vi "运维调试_氨氮.vi"() -> ()   [LabVIEW 2016, in "斯坦道氨氮.lvlib"]
uses:
  <vilib>/Utility/miscctls.llb/LVPointTypeDef.ctl
  <vilib>/Utility/config.llb/NI_LVConfig.lvlib
  <vilib>/ptbypt/NI_PtbyPt.lvlib
panel:
  in  "模块启用":bool
  in  "串口设置":bool
  in  "备用系数一键写入":bool
  in  "公式一键写入":bool
  in  "流程路径":path=path "C:/Users/STD/Documents/斯坦道流程文件/流程.xml"
  in  "曲线模型":cluster{"X^2":dbl, "X":dbl, "B":dbl}(xcontrol)
  out "字符串":string
  in  "质控参数设置":bool
  in  "自动测试量程配置":T1
  out "温度2":sgl
  out "温度1":sgl
  out "ADC":sgl
  out "固件版本号":string
  in  "数组":string[](array[string])
  in  "备用系数写入":bool
  in  "备用系数读取":bool
  in  "备用系数":T2
  in  "量程切换阈值写入":bool
  in  "量程切换阈值读取":bool
  in  "量程切换阈值":cluster{"阈值":dbl, "标液浓度":dbl}
  in  "参数下拉列表":enum16{"总磷", "总氮", "氨氮"}(ring)=enum."氨氮"
  in  "量程下拉列表":enum16{"低量程", "高量程"}(ring)
  in  "测量模式下拉列表":enum16{"水样测量", "零点核查", "跨度核查", "标样核查", "加标回收"}(ring)
  in  "公式":cluster{"X^2":dbl, "X":dbl, "b":dbl}
  in  "写公式":bool
  in  "读公式":bool
  in  "返回":bool
  in  "设置":bool
  out "序列号":string="序列号"
  out "测量数据":T3(xcontrol)
  out "集成报警信息":string
  out "定时启动":bool
  out "运行状态":T4(xcontrol)
  in  "停止":bool
  in  "手动启动":bool
  in  "单步测试":bool
  in  "总磷氨氮调试":u16[](xcontrol)
  out "F3":sgl format="%#.6f"
  out "F2":sgl format="%#.6f"
  out "F1":sgl format="%#.6f"
  out "F0":sgl format="%#.6f"
  out "多列列表框":i32(listbox)
  # "参数设置"
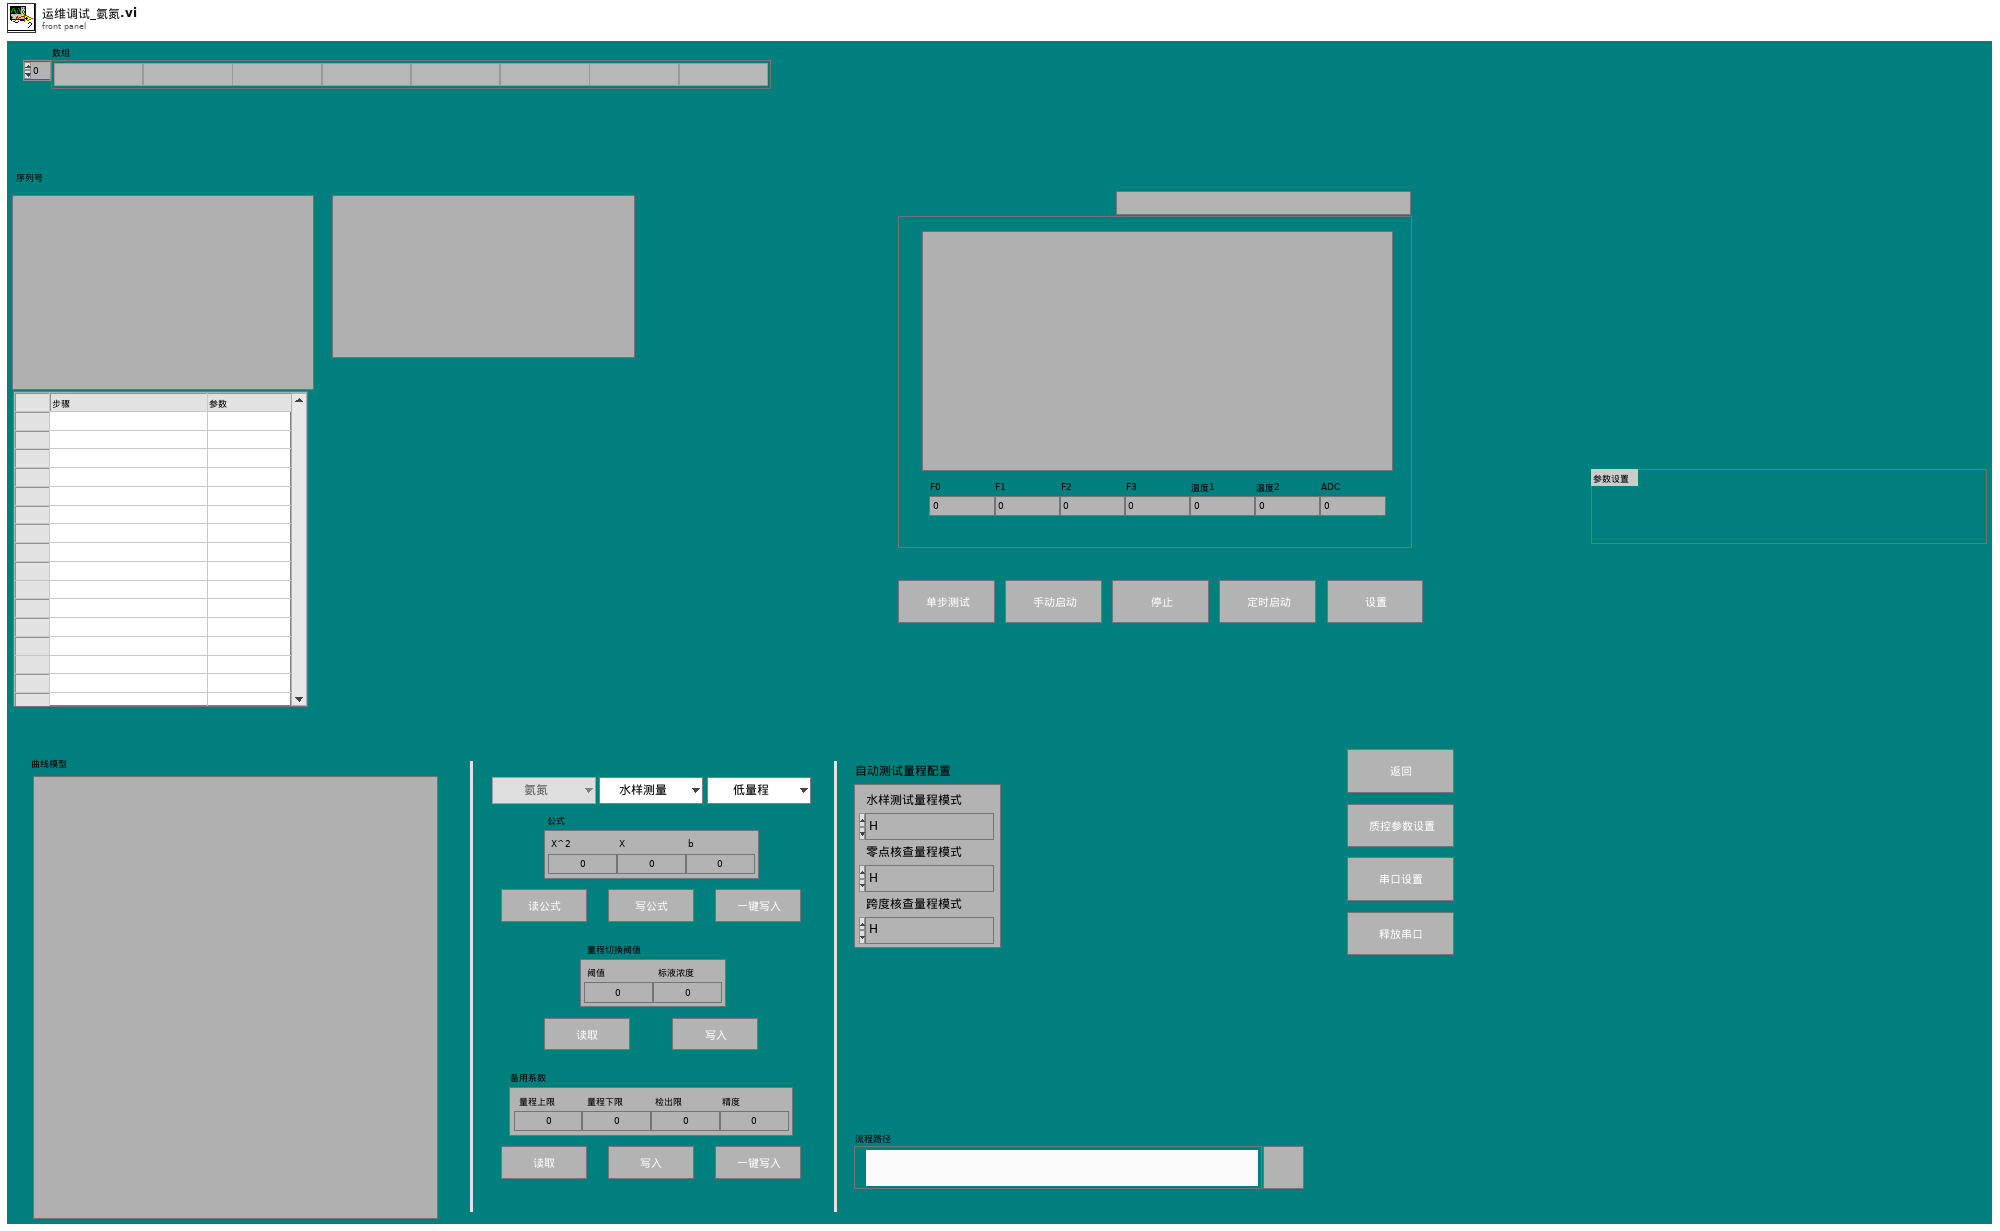
[diagram p1: front panel]
types:
  T1 = cluster{"水样测试量程模式":enum16{"H", "L", "AUTO"}, "空白核查量程模式":enum16{"H", "L", "AUTO"}, "跨度核查量程模式":enum16{"H", "L", "AUTO"}}
  T2 = cluster{"量程上限":dbl, "量程下限":dbl, "检出限":dbl, "精度":dbl}
  T3 = cluster{"flowid":u16, "测量精度":u16, "测量数据区":cluster{"因子编码":u32, "单位":u16, "标样参考值":sgl, "水样数据时间":timestamp, "水样实测值":sgl, "水样数据标识":string, "标样数据时间":timestamp, "标样实测值":sgl, "标样数据标识":string, "空白数据时间":timestamp, "空白实测值":sgl, "空白数据标识":string, "零点核查数据时间":timestamp, "零点核查实测值":sgl, "零点核查数据标识":string, "跨度核查数据时间":timestamp, "跨度核查实测值":sgl, "跨度核查数据标识":string, "加标回收数据时间":timestamp, "加标回收实测值":sgl, "加标回收数据标识":string, "平行样数据时间":timestamp, "平行样实测值":sgl, "平行样数据标识":string, "F0":sgl, "F1":sgl, "F2":sgl, "F3":sgl, "F4":sgl, "F5":sgl, "F6":sgl, "F7":sgl, "温度":sgl, "湿度":sgl, "X值":sgl}}
  T4 = cluster{"系统时间":timestamp, "工作状态":enum16{"空闲", "水样测试", "标样核查", "零点核查", "跨度核查", "空白测试", "平行样测试", "加标回收", "空白校准", "标样校准", "初始化（清洗）"}, "测量模式":enum16{"待机", "连续模式", "周期模式", "定点模式", "受控模式", "手动模式"}, "告警代码":enum16{"无告警", "缺试剂告警", "缺水样告警", "缺蒸馏水告警", "缺标液告警", "仪表漏液告警", "标定异常告警", "超量程告警", "加热异常", "低试剂预警", "超上限告警", "超下限告警", "仪表内部其他异常", "滴定异常告警", "电极异常告警", "量程切换告警", "参数设置告警", "PH电极电位异常", "电导率电极异常", "浊度光度异常", "溶解氧电极异常", "溶解氧光强异常", "温度异常告警", "PH异常告警", "溶解氧异常告警", "电导率异常告警", "浊度异常告警", "叶绿素异常告警", "藻密度异常告警", "蓝绿藻异常告警", "ORP异常告警", "氨氮异常告警", "清洁刷异常告警", "SD卡异常告警", "蓝牙异常告警", "Wifi异常告警", "流程异常告警"}, "故障代码":enum16{"无故障", "电机故障", "温度故障", "通讯故障", "滴定故障"}, "日志代码":u16, "软件版本":u16, "F0":sgl, "F1":sgl, "F2":sgl, "F3":sgl, "T":sgl, "H":sgl, "id":u16, "flowid":u16, "量程":u16, "总磷控温温度1":sgl, "营养盐控温温度2":sgl, "ADC":sgl}
  T5 = enum16{"启动测量", "标样核查", "零点核查", "跨度核查", "空白测试", "平行样测试", "加标回收", "空白校准", "标样校准", "初始化（清洗）", "停止测试", "仪器重启", "校时", "模式设置", "测量间隔设置"}
  T6 = cluster{"控制命令":enum16{"启动测量", "标样核查", "零点核查", "跨度核查", "空白测试", "平行样测试", "加标回收", "空白校准", "标样校准", "初始化（清洗）", "停止测试", "仪器重启", "校时", "模式设置", "测量间隔设置"}, "周期设置类型":enum16{"定点启动", "间隔启动"}, "定时功能启用":bool, "定时间隔":dbl, "24H周期设置":bool[], "零点核查时间":u16, "跨度核查时间":u16, "质控频次":enum16{"关闭", "每天", "星期一", "星期二", "星期三", "星期四", "星期五", "星期六", "星期日"}}
  T7 = enum16{"关闭", "每天", "星期一", "星期二", "星期三", "星期四", "星期五", "星期六", "星期日"}
  T8 = typedef "LVDateTimeRec.ctl" = cluster{"秒数的小数部分":dbl, "秒":i32, "分":i32, "时":i32, "日":i32, "月":i32, "年":i32, "天数（周）":i32, "天数（年）":i32, "DST":i32}
  T9 = enum16{"空闲", "水样测试", "标样核查", "零点核查", "跨度核查", "空白测试", "平行样测试", "加标回收", "空白校准", "标样校准", "初始化（清洗）"}
  T10 = enum32{"Bad", "Idle", "Run top level", "Running"}
  T11 = typedef "LVPointTypeDef.ctl" = cluster{"Horizontal":i16, "Vertical":i16}
  T12 = cluster{"因子编码":u32, "单位":u16, "标样参考值":sgl, "水样数据时间":timestamp, "水样实测值":sgl, "水样数据标识":string, "标样数据时间":timestamp, "标样实测值":sgl, "标样数据标识":string, "空白数据时间":timestamp, "空白实测值":sgl, "空白数据标识":string, "零点核查数据时间":timestamp, "零点核查实测值":sgl, "零点核查数据标识":string, "跨度核查数据时间":timestamp, "跨度核查实测值":sgl, "跨度核查数据标识":string, "加标回收数据时间":timestamp, "加标回收实测值":sgl, "加标回收数据标识":string, "平行样数据时间":timestamp, "平行样实测值":sgl, "平行样数据标识":string, "F0":sgl, "F1":sgl, "F2":sgl, "F3":sgl, "F4":sgl, "F5":sgl, "F6":sgl, "F7":sgl, "温度":sgl, "湿度":sgl, "X值":sgl}
  T13 = typedef "NI_LVConfig.lvlib/Config Data RefNum.ctl" = refnum<k1>
  T14 = cluster{"启动模式":enum16{"跨度核查", "水样测量", "空白核查", "标样核查", "加标回收"}, "启动参数":u16, "量程":enum16{"低量程", "高量程"}}
  T15 = cluster{"时间标识":timestamp, "设备":string, "日志信息":string, "流程参数":string}
  T16 = cluster{"时间标识":timestamp, "设备":string, "日志信息":string}
  T17 = enum16{"无告警", "缺试剂告警", "缺水样告警", "缺蒸馏水告警", "缺标液告警", "仪表漏液告警", "标定异常告警", "超量程告警", "加热异常", "低试剂预警", "超上限告警", "超下限告警", "仪表内部其他异常", "滴定异常告警", "电极异常告警", "量程切换告警", "参数设置告警", "PH电极电位异常", "电导率电极异常", "浊度光度异常", "溶解氧电极异常", "溶解氧光强异常", "温度异常告警", "PH异常告警", "溶解氧异常告警", "电导率异常告警", "浊度异常告警", "叶绿素异常告警", "藻密度异常告警", "蓝绿藻异常告警", "ORP异常告警", "氨氮异常告警", "清洁刷异常告警", "SD卡异常告警", "蓝牙异常告警", "Wifi异常告警", "流程异常告警"}
  T18 = typedef "LVRowAndColumnUnsignedTypeDef.ctl" = cluster{"Row":u32, "Column":u32}
  T19 = cluster{"站号":u16, "量程切换":enum32{"H", "L", "AUTO"}, "控制命令":enum16{"启动测量", "标样核查", "零点核查", "跨度核查", "空白测试", "平行样测试", "加标回收", "空白校准", "标样校准", "初始化（清洗）", "停止测试", "仪器重启", "校时", "模式设置", "测量间隔设置"}, "模式设置":enum16{"待机", "连续模式", "周期模式", "定点模式", "受控模式", "手动模式"}, "测量间隔":u16}
  T20 = cluster{"氨氮跨度值":dbl, "氨氮零点标准液浓度":dbl, "氨氮跨度标准液浓度":dbl, "氨氮标准液标准浓度":dbl}
  T21 = cluster{"确定":bool, "跨度值":dbl, "零点标准液浓度":dbl, "跨度标准液浓度":dbl, "标准液标准浓度":dbl}
  T22 = cluster{"控制命令":enum16{"启动测量", "标样核查", "零点核查", "跨度核查", "空白测试", "平行样测试", "加标回收", "空白校准", "标样校准", "初始化（清洗）", "停止测试", "仪器重启", "校时", "模式设置", "测量间隔设置"}, "周期设置类型":enum16{"定点启动", "间隔启动"}, "定时功能启用":bool, "定时间隔":dbl, "24H周期设置":bool[], "空白核查时间":u16, "跨度核查时间":u16, "质控频次":enum16{"关闭", "每天", "星期一", "星期二", "星期三", "星期四", "星期五", "星期六", "星期日"}}
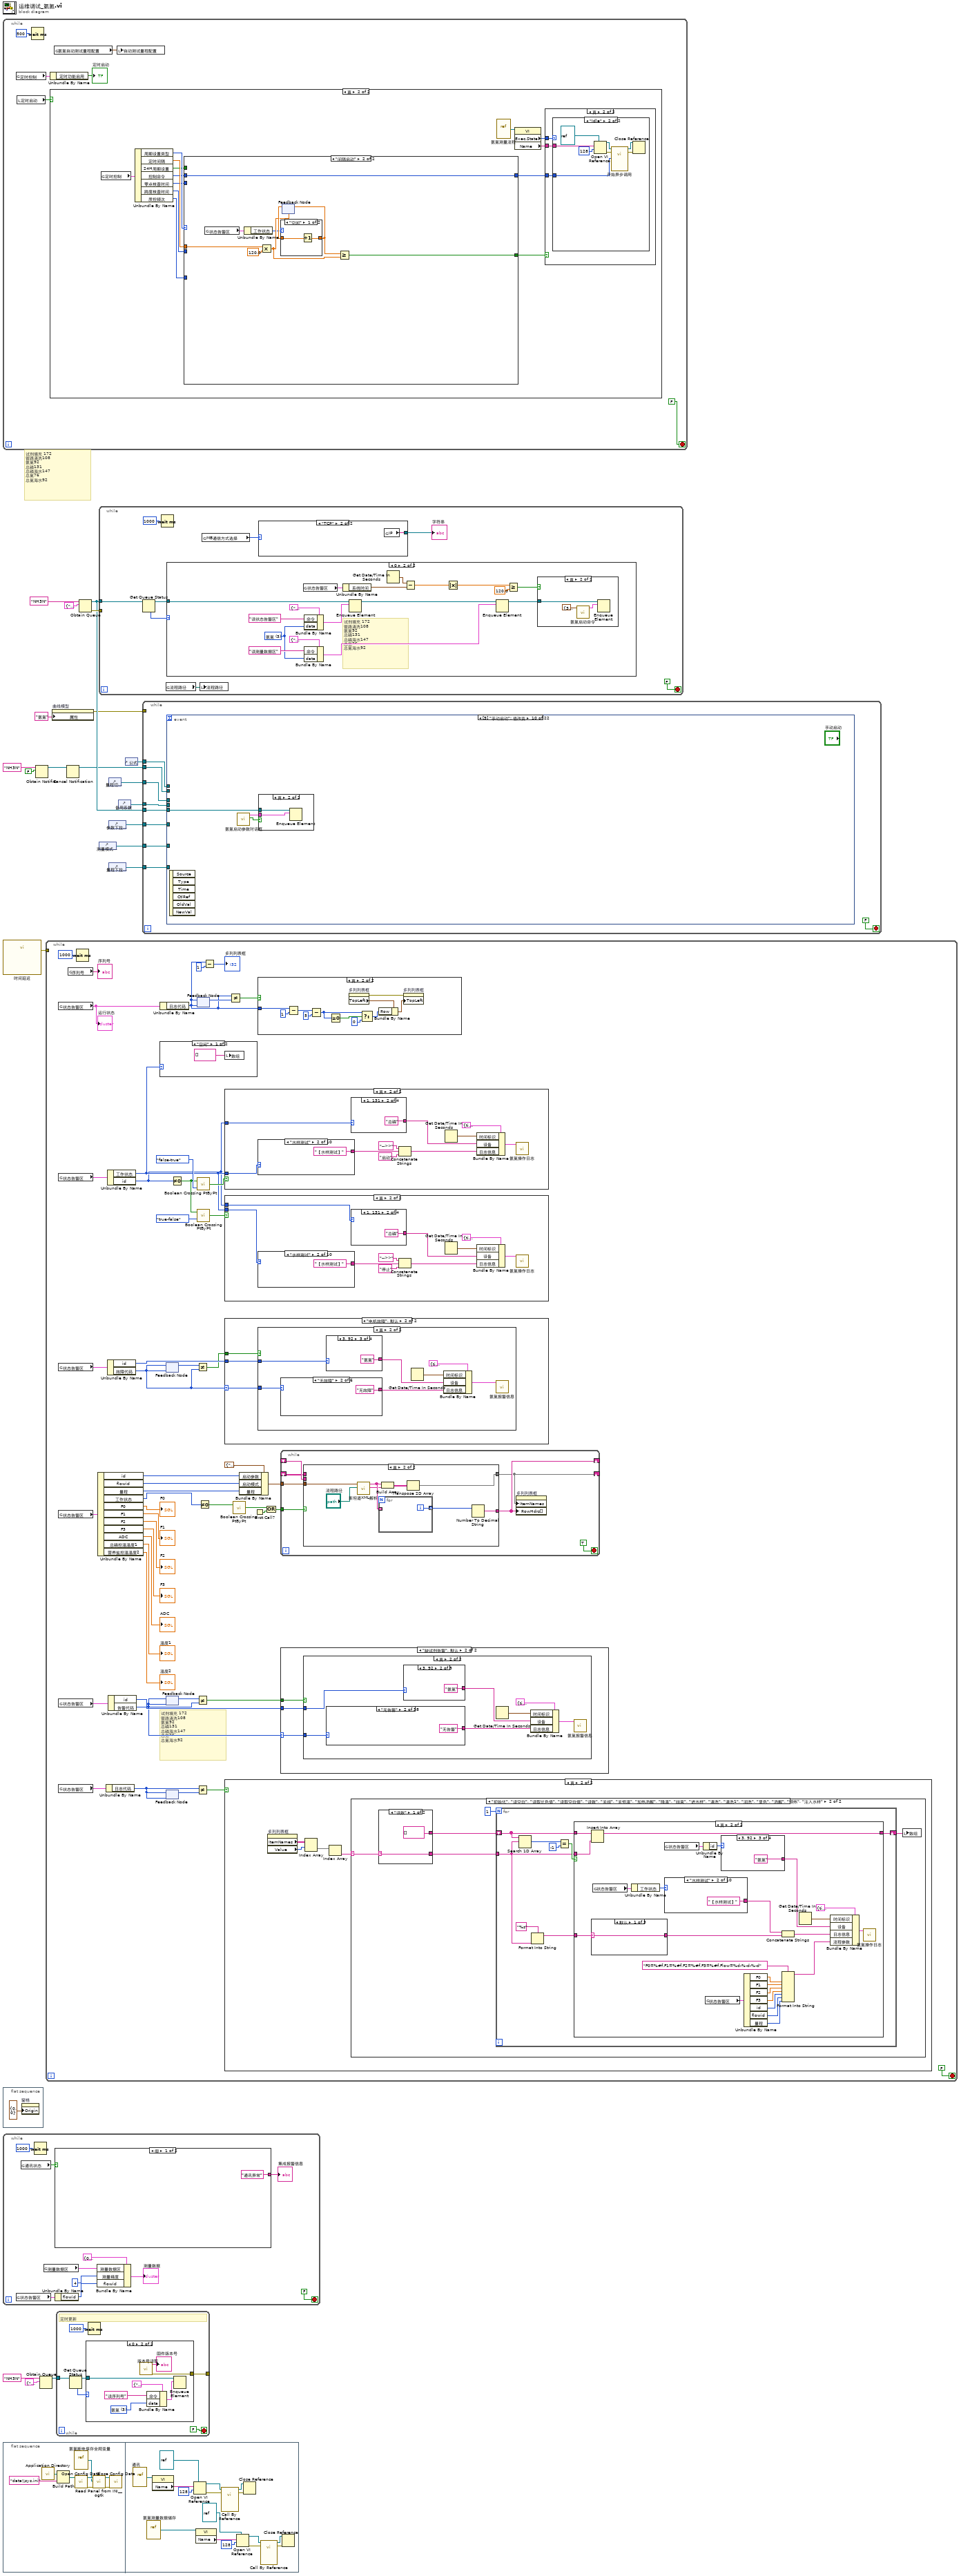
[diagram p0: block diagram]
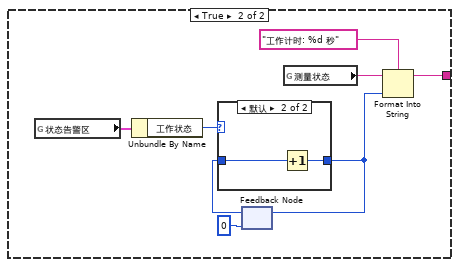
[diagram p3: hidden frame]
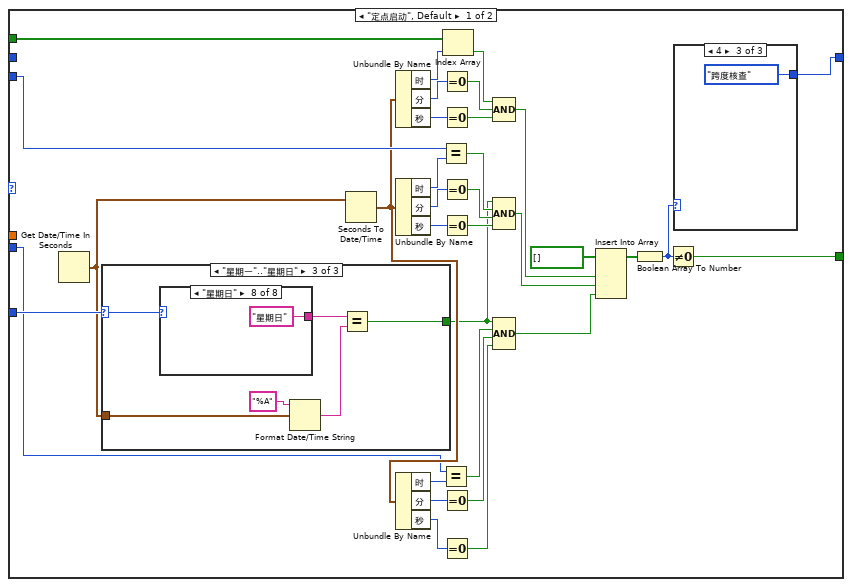
[diagram p8: hidden frame]
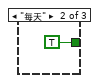
[diagram p10: hidden frame]
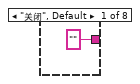
[diagram p11: hidden frame]
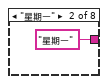
[diagram p12: hidden frame]
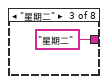
[diagram p13: hidden frame]
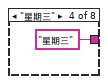
[diagram p14: hidden frame]
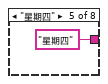
[diagram p15: hidden frame]
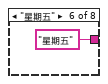
[diagram p16: hidden frame]
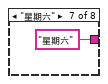
[diagram p17: hidden frame]
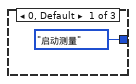
[diagram p18: hidden frame]
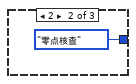
[diagram p19: hidden frame]
diagram:
  # "试剂填充 172 \n管路清洗108\n氨氮92\n总磷131\n总磷海水147\n总氮76\n总氮海水92"
  n1 = while {
    stop <- FALSE stop-if-true
    n2 = global read "氨氮断电保存全局变量.vi" "定时控制"() -> (w22:T6)
    n3 = local read "定时启动"() -> (w24:bool)
    n4 = Wait (ms)(milliseconds to wait=u32 500 ("等待时间（毫秒）")) -> ()  [unwired: 1 out]
    n5 = Unbundle By Name(w22) -> ("定时功能启用"=→"定时启动":bool)
    n6 = case shown="真" w24 {
      frame False {
      }
      frame True {
        n7 = global read "氨氮断电保存全局变量.vi" "定时控制"() -> (w39:T6)
        n8 = Unbundle By Name(w39) -> ("周期设置类型"=w38:enum16{"定点启动", "间隔启动"}, "定时间隔"=w37:dbl, "24H周期设置"=w36:bool[], "控制命令"=w31:T5, "零点核查时间"=w29:u16, "跨度核查时间"=w28:u16, "质控频次"=w27:T7)
        n9 = case shown="\"间隔启动\"" w38 {
          tunnel: w37 -> [_ w108]
          tunnel: w36 -> [w74 _]
          tunnel: [w52 w106] -> w35
          tunnel: w31 -> [_ w104]
          tunnel: [w78 w104] -> w30
          tunnel: w27 -> [w77 _]
          tunnel: w29 -> [w70 _]
          tunnel: w28 -> [w59 _]
          frame "定点启动", Default {
            n10 = Get Date/Time In Seconds() -> (seconds since 1Jan1904=w76:timestamp)
            n11 = case shown="\"星期一\"..\"星期日\"" w77 {
              selector: w77 -> [_ _ w88]
              tunnel: w76 -> [_ _ w89]
              tunnel: [_ TRUE w85] -> w58
              frame "关闭", Default {
              }
              frame "每天" {
              }
              frame "星期一".."星期日" {
                n12 = case shown="\"星期日\"" w88 {
                  tunnel: ["" ("时间格式字符串(%c)") "星期一" ("时间格式字符串(%c)") "星期二" ("时间格式字符串(%c)") "星期三" ("时间格式字符串(%c)") "星期四" ("时间格式字符串(%c)") "星期五" ("时间格式字符串(%c)") "星期六" ("时间格式字符串(%c)") "星期日" ("时间格式字符串(%c)")] -> w87
                  frame "关闭", Default {
                  }
                  frame "星期一" {
                  }
                  frame "星期二" {
                  }
                  frame "星期三" {
                  }
                  frame "星期四" {
                  }
                  frame "星期五" {
                  }
                  frame "星期六" {
                  }
                  frame "星期日" {
                  }
                }
                n13 = Format Date/Time String(time format string (%c)="%A" ("时间格式字符串(%c)"), seconds (now)=w89) -> (date/time string=w86:string)  [unwired: 1 in]
                n14 = Equal?(x=w87, y=w86) -> (x = y?=w85:bool)
              }
            }
            n15 = Seconds To Date/Time(time stamp (now)=w76) -> (date time rec=w60:T8)  [unwired: 1 in]
            n16 = Unbundle By Name(w60) -> ("时"=w83:i32, "分"=w81:i32, "秒"=w82:i32)
            n17 = Unbundle By Name(w60) -> ("时"=w71:i32, "分"=w73:i32, "秒"=w72:i32)
            n18 = Unbundle By Name(w60) -> ("时"=w63:i32, "分"=w61:i32, "秒"=w62:i32)
            n19 = Equal?(x=w70, y=w71) -> (x = y?=w69:bool)
            n20 = Equal?(x=w59, y=w63) -> (x = y?=w64:bool)
            n21 = Equal To 0?(x=w81) -> (x = 0?=w80:bool)
            n22 = Equal To 0?(x=w82) -> (x = 0?=w79:bool)
            n23 = Equal To 0?(x=w73) -> (x = 0?=w68:bool)
            n24 = Equal To 0?(x=w72) -> (x = 0?=w67:bool)
            n25 = Equal To 0?(x=w61) -> (x = 0?=w65:bool)
            n26 = Equal To 0?(x=w62) -> (x = 0?=w66:bool)
            n27 = Index Array(array=w74, index=w83) -> (element=w75:bool)
            n28 = Compound Arithmetic op=AND ("复合运算")(w75, w80, w79) -> (w56:bool)
            n29 = Compound Arithmetic op=AND ("复合运算")(w58, w69, w68, w67) -> (w55:bool)
            n30 = Compound Arithmetic op=AND ("复合运算")(w58, w64, w65, w66) -> (w54:bool)
            n31 = Insert Into Array(array=bool[] [], new element #1=w56, new element #2=w55, new element #3=w54) -> (w53:bool[])  [unwired: 1 in]
            n32 = Boolean Array To Number(Boolean array=w53) -> (number=w51:u32)
            n33 = Not Equal To 0?(x=w51) -> (x != 0?=w52:bool)
            n34 = case shown="4" w51 {
              tunnel: [T5."启动测量" ("控制命令") T5."零点核查" ("控制命令") T5."跨度核查" ("控制命令")] -> w78
              frame 0, Default {
              }
              frame 2 {
              }
              frame 4 {
              }
            }
          }
          frame "间隔启动" {
            n35 = global read "VAR氨氮全局变量.vi" "状态告警区"() -> (w103:T4)
            n36 = Unbundle By Name(w103) -> ("工作状态"=w102:T9)
            n37 = Multiply(x=w108, y=120.0) -> (x*y=w105:dbl)
            n38 = feedback #1(w105) -> (w110:dbl)
            n39 = case shown="\"空闲\"" w102 {
              tunnel: w110 -> [w112 _]
              tunnel: [w111 _] -> w109
              frame "空闲" {
                n40 = Increment(x=w112) -> (x+1=w111:dbl)
              }
              frame "水样测试", Default {
              }
            }
            n41 = feedback-in #1(w109) -> ()
            n42 = Greater Or Equal?(x=w109, y=w105) -> (x >= y?=w106:bool)
          }
        }
        n43 = vi-ref "氨氮测量流程.vi"() -> (w34:refnum<vi>)
        n44 = property class="VI"(reference=w34) -> ("Exec.State"=w33:T10, "Name"=w32:string)  [unwired: 1 in, 2 out]
        n45 = case shown="真" w35 {
          tunnel: w32 -> [_ w42]
          tunnel: w30 -> [_ w41]
          tunnel: w33 -> [_ w40]
          frame False {
          }
          frame True {
            n46 = case shown="\"Idle\"" w40 {
              tunnel: w42 -> [_ w46]
              tunnel: w41 -> [_ w44]
              frame "Bad", Default {
              }
              frame "Idle" {
                n47 = Open VI Reference(type specifier VI Refnum (for type only)=refnum<vi> refnum, vi path=w46, options=128 ("选项")) -> (vi reference=w47:refnum<vi>, error out=w48:errorcluster)  [unwired: 3 in]
                n48 = call-by-ref "开始异步调用"(reference=w47, error in=w48, "控制命令"=w44) -> (reference out=w49:refnum<vi>, error out=w50:errorcluster)  [unwired: 11 in]
                n49 = Close Reference(reference=w49, error in (no error)=w50) -> ()  [unwired: 1 out]
              }
            }
          }
        }
      }
    }
    n50 = global read "氨氮断电保存全局变量.vi" "氨氮自动测试量程配置"() -> (w23:T1)
    n51 = local write "自动测试量程配置"(w23) -> ()
  }
  n52 = call "时间延迟"() -> ("error out"=w10:errorcluster)  [unwired: 11 in]
  n53 = flat-sequence {
    frame #0 {
      n54 = property on="窗格" class="Pane"("Origin"=T11 {"Horizontal"=0, "Vertical"=0} ("原点")) -> ()  [unwired: 2 in, 2 out]
    }
  }
  n55 = while {
    stop <- FALSE stop-if-true
    n56 = global read "VAR氨氮全局变量.vi" "状态告警区"() -> (w119:T4)
    n57 = global read "VAR氨氮全局变量.vi" "通讯状态"() -> (w121:bool)
    n58 = Wait (ms)(milliseconds to wait=u32 1000 ("等待时间（毫秒）")) -> ()  [unwired: 1 out]
    n59 = global read "VAR氨氮全局变量.vi" "测量数据区"() -> (w114:T12)
    n60 = case shown="假" w121 {
      tunnel: ["通讯异常" ("集成报警信息") w126] -> w120
      frame False {
      }
      frame True {
        n61 = global read "VAR氨氮全局变量.vi" "状态告警区"() -> (w132:T4)
        n62 = Unbundle By Name(w132) -> ("工作状态"=w131:T9)
        n63 = feedback #2(0) -> (w129:i32)
        n64 = case shown="默认" w131 {
          tunnel: w129 -> [_ w134]
          tunnel: [_ w133] -> w127
          frame "空闲" {
          }
          frame Default {
            n65 = Increment(x=w134) -> (x+1=w133:i32)
          }
        }
        n66 = feedback-in #2(w127) -> ()
        n67 = global read "VAR氨氮全局变量.vi" "测量状态"() -> (w125:string)
        n68 = Format Into String(format string="工作计时: %d 秒" ("格式字符串"), initial string=w125, w127) -> (resulting string=w126:string)  [unwired: 1 in, 1 out]
      }
    }
    "集成报警信息" <- w120
    n69 = Unbundle By Name(w119) -> ("flowid"=w118:u16)
    n70 = Bundle By Name(cluster=T3 {"flowid"=0, "测量精度"=0, "测量数据区"={"因子编码"=0, "单位"=0, "标样参考值"=0.0, "水样数据时间"=timestamp(0 s since 1904-01-01), "水样实测值"=0.0, "水样数据标识"="", "标样数据时间"=timestamp(0 s since 1904-01-01), "标样实测值"=0.0, "标样数据标识"="", "空白数据时间"=timestamp(0 s since 1904-01-01), "空白实测值"=0.0, "空白数据标识"="", "零点核查数据时间"=timestamp(0 s since 1904-01-01), "零点核查实测值"=0.0, "零点核查数据标识"="", "跨度核查数据时间"=timestamp(0 s since 1904-01-01), "跨度核查实测值"=0.0, "跨度核查数据标识"="", "加标回收数据时间"=timestamp(0 s since 1904-01-01), "加标回收实测值"=0.0, "加标回收数据标识"="", "平行样数据时间"=timestamp(0 s since 1904-01-01), "平行样实测值"=0.0, "平行样数据标识"="", "F0"=0.0, "F1"=0.0, "F2"=0.0, "F3"=0.0, "F4"=0.0, "F5"=0.0, "F6"=0.0, "F7"=0.0, "温度"=0.0, "湿度"=0.0, "X值"=0.0}} ("总氮测量数据"), "测量数据区"=w114, "测量精度"=u16 4, "flowid"=w118) -> (→"测量数据":T3)
  }
  n71 = flat-sequence {
    frame #0 {
      n72 = call <vilib>:"Application Directory.vi"() -> ("Application Directory"=w142:path)
      n73 = Build Path(base path=w142, name or relative path="data\\sys.ini" ("名称或相对路径")) -> (appended path=w140:path)
      n74 = vi-ref "氨氮断电保存全局变量.vi"() -> (w138:refnum<vi>)
      n75 = call <vilib>:"Open Config Data.vi"("configuration file path"=w140) -> ("error out"=w136:errorcluster, "refnum"=w139:T13)  [unwired: 8 in, 1 out]
      n76 = call <userlib>:"Read Panel from INI__ogtk.vi"("error in (no error)"=w136, "VI ref"=w138, "refnum"=w139) -> ("error out"=w135:errorcluster, "refnum out"=w137:T13)  [unwired: 7 in]
      n77 = call <vilib>:"Close Config Data.vi"("error in (no error)"=w135, "refnum"=w137) -> ()  [unwired: 8 in, 2 out]
    }
    frame #1 {
      n78 = vi-ref "通讯.vi"() -> (w158:refnum<vi>)
      n79 = vi-ref "氨氮测量数据储存.vi"() -> (w150:refnum<vi>)
      n80 = property class="VI"(reference=w158) -> ("Name"=w157:string)  [unwired: 1 in, 2 out]
      n81 = Open VI Reference(type specifier VI Refnum (for type only)=refnum<vi> refnum, vi path=w157, options=128 ("选项")) -> (vi reference=w155:refnum<vi>, error out=w153:errorcluster)  [unwired: 3 in]
      n82 = property class="VI"(reference=w150) -> ("Name"=w143:string)  [unwired: 1 in, 2 out]
      n83 = call-by-ref "?"(reference=w155, error in=w153) -> (reference out=w151:refnum<vi>, error out=w152:errorcluster)  [unwired: 12 in]
      n84 = Open VI Reference(type specifier VI Refnum (for type only)=refnum<vi> refnum, vi path=w143, options=128 ("选项")) -> (vi reference=w145:refnum<vi>, error out=w147:errorcluster)  [unwired: 3 in]
      n85 = Close Reference(reference=w151, error in (no error)=w152) -> ()  [unwired: 1 out]
      n86 = call-by-ref "?"(reference=w145, error in=w147) -> (reference out=w149:refnum<vi>, error out=w148:errorcluster)  [unwired: 12 in]
      n87 = Close Reference(reference=w149, error in (no error)=w148) -> ()  [unwired: 1 out]
    }
  }
  n88 = Obtain Notifier(name (unnamed)="NH3N" ("名称（未命名）"), notification data type=FALSE) -> (notifier out=w2:refnum<notifier>)  [unwired: 2 in, 2 out]
  n89 = Obtain Queue(name (unnamed)="NH3N" ("名称（未命名）"), element data type=cluster{"命令":string, "data":variant} {"命令"="", "data"=variant}) -> (queue out=w7:refnum<queue>)  [unwired: 3 in, 2 out]
  n90 = while {
    tunnel: w10 -> [_]
    stop <- FALSE stop-if-true
    # "试剂填充 172 \n管路清洗108\n氨氮92\n总磷131\n总磷海水147\n总氮76\n总氮海水92"
    n91 = global read "VAR氨氮全局变量.vi" "状态告警区"() -> (w192:T4)
    "运行状态" <- w192
    n92 = global read "VAR氨氮全局变量.vi" "状态告警区"() -> (w179:T4)
    n93 = global read "VAR氨氮全局变量.vi" "状态告警区"() -> (w184:T4)
    n94 = global read "VAR氨氮全局变量.vi" "状态告警区"() -> (w200:T4)
    n95 = global read "VAR氨氮全局变量.vi" "状态告警区"() -> (w189:T4)
    n96 = global read "VAR氨氮全局变量.vi" "状态告警区"() -> (w177:T4)
    n97 = global read "VAR氨氮全局变量.vi" "序列号"() -> (→"序列号":string)
    n98 = Wait (ms)(milliseconds to wait=u32 1000 ("等待时间（毫秒）")) -> ()  [unwired: 1 out]
    n99 = Unbundle By Name(w200) -> ("id"=w197:u16, "flowid"=w199:u16, "量程"=w198:u16, "工作状态"=w167:T9, "F0"=→"F0":sgl, "F1"=→"F1":sgl, "F2"=→"F2":sgl, "F3"=→"F3":sgl, "ADC"=→"ADC":sgl, "总磷控温温度1"=→"温度1":sgl, "营养盐控温温度2"=→"温度2":sgl)
    n100 = Unbundle By Name(w177) -> ("日志代码"=w176:u16)
    n101 = Unbundle By Name(w179) -> ("工作状态"=w163:T9, "id"=w162:u16)
    n102 = Unbundle By Name(w184) -> ("id"=w183:u16, "故障代码"=w180:enum16{"无故障", "电机故障", "温度故障", "通讯故障", "滴定故障"})
    n103 = Unbundle By Name(w189) -> ("id"=w188:u16, "告警代码"=w185:T17)
    n104 = Unbundle By Name(w192) -> ("日志代码"=w173:u16)
    n105 = case shown="\"空闲\"" w163 {
      frame "空闲" {
        n106 = local write "数组"(string[] [] ("数组")) -> ()
      }
      frame "水样测试", Default {
      }
    }
    n107 = feedback #3(w180) -> (w181:enum16{"无故障", "电机故障", "温度故障", "通讯故障", "滴定故障"})
    n108 = feedback-in #3(w180) -> ()
    n109 = feedback #4(w185) -> (w186:T17)
    n110 = feedback-in #4(w185) -> ()
    n111 = feedback #5(w176) -> (w178:u16)
    n112 = feedback-in #5(w176) -> ()
    n113 = Not Equal To 0?(x=w162) -> (x != 0?=w160:bool)
    n114 = Not Equal?(x=w181, y=w180) -> (x != y?=w182:bool)
    n115 = Not Equal?(x=w186, y=w185) -> (x != y?=w187:bool)
    n116 = Not Equal?(x=w176, y=w178) -> (x != y?=w175:bool)
    n117 = feedback-in #6(w173) -> ()
    n118 = feedback #6(w173) -> (w205:u16)
    n119 = call <vilib>:"Boolean Crossing PtByPt.vi"("direction"=enum16{"either", "false-true", "true-false"}."false-true", "input"=w160) -> ("crossing"=w164:bool)  [unwired: 1 in]
    n120 = call <vilib>:"Boolean Crossing PtByPt.vi"("direction"=enum16{"either", "false-true", "true-false"}."true-false", "input"=w160) -> ("crossing"=w159:bool)  [unwired: 1 in]
    n121 = Not Equal To 0?(x=w167) -> (x != 0?=w202:bool)
    n122 = Subtract(x=w173, y=1) -> (x-y=→"多列列表框":i32)
    n123 = case shown="真" w164 {
      tunnel: w162 -> [_ w232]
      tunnel: w163 -> [_ w231]
      frame False {
      }
      frame True {
        n124 = case shown="\"水样测试\"" w231 {
          tunnel: [_ "【水样测试】" ("字符串") "【标样核查】" ("字符串") "【零点核查】" ("字符串") "【跨度核查】" ("字符串") "【空白测试】" ("字符串") "【平行样测试】" ("字符串") "【加标回收】" ("字符串") "【空白校准】" ("字符串") "【标样校准】" ("字符串")] -> w236
          frame "空闲", Default {
          }
          frame "水样测试" {
          }
          frame "标样核查" {
          }
          frame "零点核查" {
          }
          frame "跨度核查" {
          }
          frame "空白测试" {
          }
          frame "平行样测试" {
          }
          frame "加标回收" {
          }
          frame "空白校准" {
          }
          frame "标样校准" {
          }
        }
        n125 = case shown="1, 131" w232 {
          tunnel: [_ "总磷" ("table输入") "氨氮" ("table输入") "总氮" ("table输入")] -> w237
          frame Default {
          }
          frame 1, 131 {
          }
          frame 3, 92 {
          }
          frame 2, 76 {
          }
        }
        n126 = Concatenate Strings("-->>" ("字符串"), w236, "启动" ("字符串")) -> (w235:string)
        n127 = Get Date/Time In Seconds() -> (seconds since 1Jan1904=w238:timestamp)
        n128 = Bundle By Name(cluster=T15 {"时间标识"=timestamp(0 s since 1904-01-01), "设备"="", "日志信息"="", "流程参数"=""} ("data in"), "时间标识"=w238, "设备"=w237, "日志信息"=w235) -> (w230:T15)
        n129 = call "氨氮操作日志.vi"("data in"=w230) -> ()  [unwired: 11 in]
      }
    }
    n130 = case shown="真" w159 {
      tunnel: w162 -> [_ w210]
      tunnel: w163 -> [_ w209]
      frame False {
      }
      frame True {
        n131 = case shown="\"水样测试\"" w209 {
          tunnel: [_ "【水样测试】" ("字符串") "【标样核查】" ("字符串") "【零点核查】" ("字符串") "【跨度核查】" ("字符串") "【空白测试】" ("字符串") "【平行样测试】" ("字符串") "【加标回收】" ("字符串") "【空白校准】" ("字符串") "【标样校准】" ("字符串")] -> w214
          frame "空闲", Default {
          }
          frame "水样测试" {
          }
          frame "标样核查" {
          }
          frame "零点核查" {
          }
          frame "跨度核查" {
          }
          frame "空白测试" {
          }
          frame "平行样测试" {
          }
          frame "加标回收" {
          }
          frame "空白校准" {
          }
          frame "标样校准" {
          }
        }
        n132 = case shown="1, 131" w210 {
          tunnel: [_ "总磷" ("table输入") "氨氮" ("table输入") "总氮" ("table输入")] -> w215
          frame Default {
          }
          frame 1, 131 {
          }
          frame 3, 92 {
          }
          frame 2, 76 {
          }
        }
        n133 = Concatenate Strings("-->>" ("字符串"), w214, "停止" ("字符串")) -> (w213:string)
        n134 = Get Date/Time In Seconds() -> (seconds since 1Jan1904=w216:timestamp)
        n135 = Bundle By Name(cluster=T15 {"时间标识"=timestamp(0 s since 1904-01-01), "设备"="", "日志信息"="", "流程参数"=""} ("data in"), "时间标识"=w216, "设备"=w215, "日志信息"=w213) -> (w208:T15)
        n136 = call "氨氮操作日志.vi"("data in"=w208) -> ()  [unwired: 11 in]
      }
    }
    n137 = case shown="\"电机故障\", 默认" w180 {
      selector: w180 -> [_ w320]
      tunnel: w183 -> [_ w321]
      tunnel: w182 -> [_ w319]
      frame "无故障" {
      }
      frame "电机故障", Default {
        n138 = case shown="真" w319 {
          tunnel: w321 -> [_ w328]
          tunnel: w320 -> [_ w323]
          frame False {
          }
          frame True {
            n139 = case shown="\"无故障\"" w323 {
              selector: w323 -> [w330 _ _ _ _ _]
              tunnel: [w329 "无故障" "电机故障" "温度故障" "通讯故障" "滴定故障"] -> w322
              frame Default {
                n140 = Format Into String(format string="%d" ("格式字符串"), initial string="未知" ("工作状态"), w330) -> (resulting string=w329:string)  [unwired: 1 in, 1 out]
              }
              frame "无故障" {
              }
              frame "电机故障" {
              }
              frame "温度故障" {
              }
              frame "通讯故障" {
              }
              frame "滴定故障" {
              }
            }
            n141 = case shown="3, 92" w328 {
              tunnel: [_ "总磷" ("table输入") "氨氮" ("table输入") "总氮" ("table输入")] -> w324
              frame Default {
              }
              frame 1, 131 {
              }
              frame 3, 92 {
              }
              frame 2, 76 {
              }
            }
            n142 = Get Date/Time In Seconds() -> (seconds since 1Jan1904=w325:timestamp)
            n143 = Bundle By Name(cluster=T16 {"时间标识"=timestamp(0 s since 1904-01-01), "设备"="", "日志信息"=""} ("data in"), "时间标识"=w325, "设备"=w324, "日志信息"=w322) -> (w326:T16)
            n144 = call "氨氮报警信息.vi"("data in"=w326) -> ()  [unwired: 10 in, 1 out]
          }
        }
      }
    }
    n145 = case shown="真" w175 {
      frame False {
      }
      frame True {
        n146 = property on="多列列表框" class="MCListbox (严格)"() -> ("ItemNames"=w255:string[][], "Value"=w256:i32)  [unwired: 2 in, 2 out]
        n147 = Index Array(array=w255, index (row)=w256) -> (element=w254:string[])  [unwired: 1 in]
        n148 = Index Array(array=w254) -> (element=w253:string)  [unwired: 1 in]
        n149 = case shown="\"初始化\", \"读空白\", \"读取比色值\", \"读取空白值\", \"读数\", \"关阀\", \"关恒温\", \"加热消解\", \"降温\", \"结束\", \"进水样\", \"清洗\", \"清洗1\", \"润洗\", \"显色\", \"消解\", \"预热\", \"注入水样\"" w253 {
          selector: w253 -> [_ w259]
          frame Default {
          }
          frame "初始化", "读空白", "读取比色值", "读取空白值", "读数", "关阀", "关恒温", "加热消解", "降温", "结束", "进水样", "清洗", "清洗1", "润洗", "显色", "消解", "预热", "注入水样" {
            n150 = case shown="\"读数\"" w259 {
              selector: w259 -> [w263 w265]
              tunnel: [w263 w265] -> w258
              tunnel: [string[] [] ("数组") "数组"] -> w257
              frame "读数" {
              }
              frame Default {
              }
            }
            n151 = for {
              N: 1 -> [_]
              tunnel: w258 -> [w267]
              shift-right: [w266] -> w260
              shift-left: w257 -> [w268]
              n152 = Search 1D Array(1D array=w268, element=w267) -> (index of element=w271:i32)  [unwired: 1 in]
              n153 = Format Into String(format string="%s" ("格式字符串"), w267) -> (resulting string=w272:string)  [unwired: 2 in, 1 out]
              n154 = Equal?(x=w271, y=-1) -> (x = y?=w269:bool)
              n155 = case shown="真" w269 {
                tunnel: w272 -> [_ w280]
                tunnel: w268 -> [w274 w284]
                tunnel: w267 -> [_ w283]
                tunnel: [w274 w282] -> w266
                frame False {
                }
                frame True {
                  n156 = Insert Into Array(array=w284, new element=w283) -> (w282:string[])  [unwired: 1 in]
                  n157 = case shown="默认" w280 {
                    selector: w280 -> [w309 w312 w315]
                    tunnel: [w309 w311 w314] -> w279
                    frame Default {
                    }
                    frame "初始化" {
                      n158 = Concatenate Strings("-->>" ("字符串"), w312) -> (w311:string)
                    }
                    frame "结束" {
                      n159 = Concatenate Strings("-->>" ("字符串"), w315) -> (w314:string)
                    }
                  }
                  n160 = global read "VAR氨氮全局变量.vi" "状态告警区"() -> (w278:T4)
                  n161 = Unbundle By Name(w278) -> ("工作状态"=w277:T9)
                  n162 = global read "VAR氨氮全局变量.vi" "状态告警区"() -> (w299:T4)
                  n163 = case shown="\"水样测试\"" w277 {
                    tunnel: [_ "【水样测试】" ("字符串") "【标样核查】" ("字符串") "【零点核查】" ("字符串") "【跨度核查】" ("字符串") "【空白测试】" ("字符串") "【平行样测试】" ("字符串") "【加标回收】" ("字符串") "【空白校准】" ("字符串") "【标样校准】" ("字符串")] -> w275
                    frame "空闲", Default {
                    }
                    frame "水样测试" {
                    }
                    frame "标样核查" {
                    }
                    frame "零点核查" {
                    }
                    frame "跨度核查" {
                    }
                    frame "空白测试" {
                    }
                    frame "平行样测试" {
                    }
                    frame "加标回收" {
                    }
                    frame "空白校准" {
                    }
                    frame "标样校准" {
                    }
                  }
                  n164 = Unbundle By Name(w299) -> ("id"=w298:u16)
                  n165 = global read "VAR氨氮全局变量.vi" "状态告警区"() -> (w294:T4)
                  n166 = case shown="3, 92" w298 {
                    tunnel: [_ "总磷" ("table输入") "氨氮" ("table输入") "总氮" ("table输入")] -> w296
                    frame Default {
                    }
                    frame 1, 131 {
                    }
                    frame 3, 92 {
                    }
                    frame 2, 76 {
                    }
                  }
                  n167 = Unbundle By Name(w294) -> ("F0"=w291:sgl, "F1"=w290:sgl, "F2"=w289:sgl, "F3"=w288:sgl, "id"=w287:u16, "flowid"=w286:u16, "量程"=w285:u16)
                  n168 = Concatenate Strings(w275, w279) -> (w276:string)
                  n169 = Format Into String(format string="F0=%#f,F1=%#f,F2=%#f,F3=%#f,Flow=%d-%-d-%-d" ("格式字符串"), w291, w290, w289, w288, w287, w286, w285) -> (resulting string=w292:string)  [unwired: 2 in, 1 out]
                  n170 = Get Date/Time In Seconds() -> (seconds since 1Jan1904=w295:timestamp)
                  n171 = Bundle By Name(cluster=T15 {"时间标识"=timestamp(0 s since 1904-01-01), "设备"="", "日志信息"="", "流程参数"=""} ("data in"), "时间标识"=w295, "设备"=w296, "日志信息"=w276, "流程参数"=w292) -> (w297:T15)
                  n172 = call "氨氮操作日志.vi"("data in"=w297) -> ()  [unwired: 11 in]
                }
              }
            }
            n173 = local write "数组"(w260) -> ()
          }
        }
      }
    }
    n174 = Not Equal?(x=w173, y=w205) -> (x != y?=w204:bool)
    n175 = call <vilib>:"Boolean Crossing PtByPt.vi"("input"=w202) -> ("crossing"=w166:bool)  [unwired: 2 in]
    n176 = Bundle By Name(cluster=T14 {"启动模式"=enum."跨度核查", "启动参数"=1, "量程"=enum."低量程"} ("参数簇"), "启动参数"=w197, "启动模式"=w199, "量程"=w198) -> (w191:T14)
    n177 = First Call?() -> (First Call?: T/F=w203:bool)
    n178 = case shown="真" w204 {
      tunnel: w173 -> [_ w415]
      frame False {
      }
      frame True {
        n179 = Subtract(x=w415, y=1) -> (x-y=w413:i32)
        n180 = Subtract(x=w413, y=5) -> (x-y=w417:i32)
        n181 = Greater Or Equal To 0?(x=w417) -> (x >= 0?=w416:bool)
        n182 = property on="多列列表框" class="MCListbox (严格)"() -> (error out=w421:errorcluster, "TopLeft"=w422:T18)  [unwired: 2 in, 1 out]
        n183 = Select(t=w417, s=w416, f=0) -> (s? t:f=w418:i32)
        n184 = Bundle By Name(cluster=w422, "Row"=w418) -> (w423:T18)
        n185 = property on="多列列表框" class="MCListbox (严格)"(error in=w421, "TopLeft"=w423) -> ()  [unwired: 1 in, 2 out]
      }
    }
    n186 = Or(x=w166, y=w203) -> (x .or. y?=w201:bool)
    n187 = while {
      tunnel: w201 -> [w401]
      tunnel: w191 -> [w400]
      shift-right: [w395] -> _
      shift-left: _ -> [w397]
      shift-right: [w396] -> _
      shift-left: _ -> [w398]
      stop <- TRUE stop-if-true
      n188 = case shown="真" w401 {
        tunnel: [w403 w411] -> w396
        tunnel: [w402 w410] -> w395
        tunnel: w400 -> [_ w405]
        tunnel: w398 -> [w403 _]
        tunnel: w397 -> [w402 _]
        frame False {
        }
        frame True {
          n189 = call "斯坦道XML解析.vi"("添加的路径"="流程路径", "参数簇"=w405) -> ("步骤时间"=w406:string[], "步骤名"=w408:string[])  [unwired: 8 in]
          n190 = for {
            tunnel: w408 -> [_] mode=indexing
            tunnel: [w412] -> w409 mode=indexing
            i -> [w412]
          }
          n191 = Build Array(w408, w406) -> (w407:string[][])
          n192 = Transpose 2D Array(2D array=w407) -> (transposed array=w410:string[][])
          n193 = Number To Decimal String(number=w409) -> (decimal integer string=w411:string[])  [unwired: 1 in]
        }
      }
      n194 = property on="多列列表框" class="MCListbox (严格)"("ItemNames"=w395, "RowHdrs[]"=w396) -> ()  [unwired: 2 in, 2 out]
    }
    n195 = case shown="\"缺试剂告警\", 默认" w185 {
      selector: w185 -> [_ w342]
      tunnel: w188 -> [_ w343]
      tunnel: w187 -> [_ w341]
      frame "无告警" {
      }
      frame "缺试剂告警", Default {
        n196 = case shown="真" w341 {
          tunnel: w343 -> [_ w350]
          tunnel: w342 -> [_ w344]
          frame False {
          }
          frame True {
            n197 = case shown="\"无告警\"" w344 {
              selector: w344 -> [w352 _ _ _ _ _ _ _ _ _ _ _ _ _ _ _ _ _ _ _ _ _ _ _ _ _ _ _ _ _ _ _ _ _ _ _ _ _]
              tunnel: [w351 "无告警" "缺试剂告警" "缺水样告警" "缺蒸馏水告警" "缺标液告警" "仪表漏液告警" "标定异常告警" "超量程告警" "加热异常" "低试剂预警" "超上限告警" "超下限告警" "仪表内部其他异常" "滴定异常告警" "电极异常告警" "量程切换告警" "参数设置告警" "PH电极电位异常" "电导率电极异常" "浊度光度异常" "溶解氧电极异常" "溶解氧光强异常" "温度异常告警" "PH异常告警" "溶解氧异常告警" "电导率异常告警" "浊度异常告警" "叶绿素异常告警" "藻密度异常告警" "蓝绿藻异常告警" "ORP异常告警" "氨氮异常告警" "清洁刷异常告警" "SD卡异常告警" "蓝牙异常告警" "WiFi异常告警" "流程异常告警"] -> w345
              frame Default {
                n198 = Format Into String(format string="%d" ("格式字符串"), initial string="未知" ("工作状态"), w352) -> (resulting string=w351:string)  [unwired: 1 in, 1 out]
              }
              frame "无告警" {
              }
              frame "缺试剂告警" {
              }
              frame "缺水样告警" {
              }
              frame "缺蒸馏水告警" {
              }
              frame "缺标液告警" {
              }
              frame "仪表漏液告警" {
              }
              frame "标定异常告警" {
              }
              frame "超量程告警" {
              }
              frame "加热异常" {
              }
              frame "低试剂预警" {
              }
              frame "超上限告警" {
              }
              frame "超下限告警" {
              }
              frame "仪表内部其他异常" {
              }
              frame "滴定异常告警" {
              }
              frame "电极异常告警" {
              }
              frame "量程切换告警" {
              }
              frame "参数设置告警" {
              }
              frame "PH电极电位异常" {
              }
              frame "电导率电极异常" {
              }
              frame "浊度光度异常" {
              }
              frame "溶解氧电极异常" {
              }
              frame "溶解氧光强异常" {
              }
              frame "温度异常告警" {
              }
              frame "PH异常告警" {
              }
              frame "溶解氧异常告警" {
              }
              frame "电导率异常告警" {
              }
              frame "浊度异常告警" {
              }
              frame "叶绿素异常告警" {
              }
              frame "藻密度异常告警" {
              }
              frame "蓝绿藻异常告警" {
              }
              frame "ORP异常告警" {
              }
              frame "氨氮异常告警" {
              }
              frame "清洁刷异常告警" {
              }
              frame "SD卡异常告警" {
              }
              frame "蓝牙异常告警" {
              }
              frame "Wifi异常告警" {
              }
              frame "流程异常告警" {
              }
            }
            n199 = case shown="3, 92" w350 {
              tunnel: ["总磷" ("table输入") "氨氮" ("table输入") "总氮" ("table输入")] -> w346
              frame 1, 131 {
              }
              frame 3, 92 {
              }
              frame 2, 76, Default {
              }
            }
            n200 = Get Date/Time In Seconds() -> (seconds since 1Jan1904=w347:timestamp)
            n201 = Bundle By Name(cluster=T16 {"时间标识"=timestamp(0 s since 1904-01-01), "设备"="", "日志信息"=""} ("data in"), "时间标识"=w347, "设备"=w346, "日志信息"=w345) -> (w348:T16)
            n202 = call "氨氮报警信息.vi"("data in"=w348) -> ()  [unwired: 10 in, 1 out]
          }
        }
      }
    }
  }
  n203 = property on="曲线模型" class="曲线模型 (严格)"("属性"="氨氮" ("调用模块名称属性")) -> (error out=w5:errorcluster)  [unwired: 2 in, 1 out]
  n204 = while {
    tunnel: w7 -> [w428]
    tunnel: [w426] -> _
    stop <- FALSE stop-if-true
    # "定时更新"
    n205 = Get Queue Status(queue=w428) -> (queue out=w425:refnum<queue>, # elements in queue=w424:i32)  [unwired: 2 in, 6 out]
    n206 = case shown="0" w424 {
      tunnel: [_ w431] -> w426
      tunnel: w425 -> [_ w430]
      frame Default {
      }
      frame 0 {
        w434 = u16 3 items=["总磷"=1, "氨氮"=3] ("站号")
        n207 = call "版本号读取.vi"() -> ("error out"=w431:errorcluster, "固件版本号"=→"固件版本号":string)  [unwired: 10 in]
        n208 = Bundle By Name(cluster=cluster{"命令":string, "data":variant} {"命令"="", "data"=variant} ("元素"), "命令"="读序列号", "data"=w434) -> (w433:cluster{"命令":string, "data":variant})
        n209 = Enqueue Element(queue=w430, element=w433) -> ()  [unwired: 2 in, 3 out]
      }
    }
    n210 = Wait (ms)(milliseconds to wait=u32 1000 ("等待时间（毫秒）")) -> ()  [unwired: 1 out]
  }
  n211 = Cancel Notification(0:w2) -> (8:w1:refnum<notifier>)  [unwired: 1 in, 2 out]
  n212 = Obtain Queue(name (unnamed)="NH3N" ("名称（未命名）"), element data type=cluster{"命令":string, "data":variant} {"命令"="", "data"=variant}) -> (queue out=w17:refnum<queue>, error out=w18:errorcluster)  [unwired: 3 in, 1 out]
  n213 = while {
    tunnel: w17 -> [w442]
    tunnel: w18 -> [_]
    stop <- FALSE stop-if-true
    n214 = Get Queue Status(queue=w442) -> (queue out=w438:refnum<queue>, # elements in queue=w437:i32)  [unwired: 2 in, 6 out]
    n215 = Wait (ms)(milliseconds to wait=u32 1000 ("等待时间（毫秒）")) -> ()  [unwired: 1 out]
    n216 = global read "氨氮断电保存全局变量.vi" "流程路径"() -> (w441:path)
    n217 = case shown="0" w437 {
      tunnel: w438 -> [_ w445]
      frame Default {
      }
      frame 0 {
        w454 = u16 3 items=["总磷"=1, "氨氮"=3] ("站号")
        # "试剂填充 172 \n管路清洗108\n氨氮92\n总磷131\n总磷海水147\n总氮76\n总氮海水92"
        n218 = global read "VAR氨氮全局变量.vi" "状态告警区"() -> (w446:T4)
        n219 = Bundle By Name(cluster=cluster{"命令":string, "data":variant} {"命令"="", "data"=variant} ("元素"), "命令"="读状态告警区", "data"=w454) -> (w460:cluster{"命令":string, "data":variant})
        n220 = Bundle By Name(cluster=cluster{"命令":string, "data":variant} {"命令"="", "data"=variant} ("元素"), "命令"="读测量数据区", "data"=w454) -> (w457:cluster{"命令":string, "data":variant})
        n221 = Unbundle By Name(w446) -> ("系统时间"=w453:timestamp)
        n222 = Enqueue Element(queue=w445, element=w460) -> (queue out=w455:refnum<queue>)  [unwired: 2 in, 2 out]
        n223 = Get Date/Time In Seconds() -> (seconds since 1Jan1904=w452:timestamp)
        n224 = Subtract(x=w452, y=w453) -> (x-y=w451:dbl)
        n225 = Absolute Value(x=w451) -> (abs(x)=w450:dbl)
        n226 = Enqueue Element(queue=w455, element=w457) -> (queue out=w447:refnum<queue>)  [unwired: 2 in, 2 out]
        n227 = Greater Or Equal?(x=w450, y=120.0) -> (x >= y?=w448:bool)
        n228 = case shown="真" w448 {
          tunnel: w447 -> [_ w463]
          frame False {
          }
          frame True {
            n229 = call "氨氮启动命令.vi"("参数"=T19 {"站号"=3, "量程切换"=enum."AUTO", "控制命令"=enum."校时", "模式设置"=enum."待机", "测量间隔"=0}) -> ("启动命令"=w462:cluster{"命令":string, "data":variant})  [unwired: 10 in]
            n230 = Enqueue Element(queue=w463, element=w462) -> ()  [unwired: 2 in, 3 out]
          }
        }
      }
    }
    n231 = local write "流程路径"(w441) -> ()
    n232 = global read "氨氮断电保存全局变量.vi" "MB通信方式选择"() -> (w439:enum16{"串口", "TCP"})
    n233 = case shown="\"TCP\"" w439 {
      tunnel: [w465 w466] -> w440
      frame "串口", Default {
        n234 = global read "氨氮断电保存全局变量.vi" "VISA Resource"() -> (w465:refnum<visa-resource-name>)
      }
      frame "TCP" {
        n235 = global read "氨氮断电保存全局变量.vi" "IP"() -> (w466:string)
      }
    }
    "字符串" <- w440
  }
  n236 = control-ref of="测量模式下拉列表"() -> (w14:refnum<vi>)
  n237 = control-ref of="量程切换阈值"() -> (w12:refnum<vi>)
  n238 = control-ref of="参数下拉列表"() -> (w15:refnum<vi>)
  n239 = control-ref of="量程下拉列表"() -> (w16:refnum<vi>)
  n240 = control-ref of="备用系数"() -> (w11:refnum<vi>)
  n241 = control-ref of="公式"() -> (w13:refnum<vi>)
  n242 = while {
    tunnel: w17 -> [w474]
    tunnel: w16 -> [w473]
    tunnel: w15 -> [w472]
    tunnel: w14 -> [w471]
    tunnel: w13 -> [w470]
    tunnel: w12 -> [w469]
    tunnel: w11 -> [w468]
    tunnel: w5 -> [_]
    tunnel: w1 -> [w467]
    stop <- FALSE stop-if-true
    n243 = event shown="[9] \"手动启动\": 值改变" {
      selector: _ -> [_ _ _ _ _ _ _ _ _ _ _ _ _ _ _ _ _ _ _ _ _ _]
      dyn-events: _ -> [_ _ _ _ _ _ _ _ _ _ _ _ _ _ _ _ _ _ _ _ _ _]
      timeout: _ -> [_ _ _ _ _ _ _ _ _ _ _ _ _ _ _ _ _ _ _ _ _ _]
      tunnel: w474 -> [_ w485 w513 _ _ _ _ _ _ w580 _ w605 w612 _ _ _ _ _ _ _ _ _]
      tunnel: w473 -> [_ _ _ _ _ _ _ _ _ _ _ _ _ _ _ _ w628 _ w648 w657 w663 w675]
      tunnel: w472 -> [_ _ _ _ _ _ _ _ _ _ _ _ _ _ _ _ w626 _ w646 w659 w671 w682]
      tunnel: w471 -> [_ _ _ _ _ _ _ _ _ _ _ _ _ _ _ _ w627 _ w647 w658 w665 w677]
      tunnel: w470 -> [_ _ _ _ _ _ _ _ _ _ _ _ _ _ _ _ w622 _ _ _ _ _]
      tunnel: w469 -> [_ _ _ _ _ _ _ _ _ _ _ _ _ _ _ _ _ _ w642 _ _ _]
      tunnel: w468 -> [_ _ _ _ _ _ _ _ _ _ _ _ _ _ _ _ _ _ _ _ w669 _]
      tunnel: w467 -> [_ _ _ _ _ _ _ _ _ _ _ _ w607 _ _ _ _ _ _ _ _ _]
      event Timeout {
        n244 = event-data() -> ()  [unwired: 1 in, 3 out]
      }
      event "串口设置": Value Change {
        n245 = event-data() -> ()  [unwired: 1 in, 6 out]
        n246 = global read "氨氮断电保存全局变量.vi" "MB通信方式选择"() -> (w476:enum16{"串口", "TCP"})
        n247 = global read "氨氮断电保存全局变量.vi" "VISA Resource"() -> (w482:refnum<visa-resource-name>)
        n248 = global read "氨氮断电保存全局变量.vi" "PORT"() -> (w480:string)
        n249 = global read "氨氮断电保存全局变量.vi" "IP"() -> (w481:string)
        n250 = call "串口配置.vi"("PORT"=w480, "IP"=w481, "MB通信方式选择"=w476, "请选择串口:"=w482) -> ("PORT 2"=w478:string, "IP 2"=w479:string, "确认 2"=w483:bool, "VISA资源名称 2"=w484:refnum<visa-resource-name>, "MB通信方式选择 2"=w477:enum16{"串口", "TCP"})  [unwired: 3 in]
        n251 = case shown="真" w483 {
          tunnel: w484 -> [_ w490]
          tunnel: w485 -> [_ w489]
          tunnel: w479 -> [_ w488]
          tunnel: w478 -> [_ w487]
          tunnel: w477 -> [_ w486]
          frame False {
          }
          frame True {
            n252 = flat-sequence {
              tunnel: w490 -> [w495]
              tunnel: w489 -> [w496]
              tunnel: w488 -> [w494]
              tunnel: w487 -> [w493]
              tunnel: w486 -> [w492]
              frame #0 {
                n253 = global write "氨氮断电保存全局变量.vi" "IP"(w494) -> ()
                n254 = global write "氨氮断电保存全局变量.vi" "PORT"(w493) -> ()
                n255 = global write "氨氮断电保存全局变量.vi" "VISA Resource"(w495) -> ()
                n256 = global write "氨氮断电保存全局变量.vi" "MB通信方式选择"(w492) -> ()
                n257 = Flush Queue(queue=w496) -> (queue out=w491:refnum<queue>)  [unwired: 1 in, 2 out]
                n258 = Enqueue Element(queue=w491, element=cluster{"命令":string, "data":variant} {"命令"="启用模块", "data"=variant} ("元素")) -> ()  [unwired: 2 in, 3 out]
              }
              frame #1 {
                n259 = call <vilib>:"Application Directory.vi"() -> ("Application Directory"=w511:path)
                n260 = Build Path(base path=w511, name or relative path="data\\sys.ini" ("名称或相对路径")) -> (appended path=w509:path)
                n261 = call <vilib>:"Open Config Data.vi"("configuration file path"=w509) -> ("error out"=w505:errorcluster, "refnum"=w508:T13)  [unwired: 8 in, 1 out]
                n262 = vi-ref "氨氮断电保存全局变量.vi"() -> (w507:refnum<vi>)
                n263 = call <userlib>:"Write Panel to INI__ogtk.vi"("error in (no error)"=w505, "VI ref"=w507, "refnum"=w508) -> ("error out"=w504:errorcluster, "refnum out"=w506:T13)  [unwired: 7 in]
                n264 = call <vilib>:"Close Config Data.vi"("error in (no error)"=w504, "refnum"=w506) -> ("error out"=w499:errorcluster, "file path"=w498:path)  [unwired: 8 in]
                n265 = Open/Create/Replace File(file path (use dialog)=w498, error in=w499) -> (refnum out=w502:refnum<file>, error out=w503:errorcluster)  [unwired: 4 in, 1 out]
                n266 = Flush File(refnum=w502, error in=w503) -> (refnum out=w501:refnum<file>, error out=w500:errorcluster)
                n267 = Close File(refnum=w501, error in=w500) -> ()  [unwired: 2 out]
              }
            }
          }
        }
      }
      event "模块启用": Value Change {
        n268 = event-data() -> ("OldVal"=w514:bool)  [unwired: 1 in, 5 out]
        n269 = Flush Queue(queue=w513) -> (queue out=w512:refnum<queue>)  [unwired: 1 in, 2 out]
        n270 = case shown="假" w514 {
          tunnel: w512 -> [w515 w517]
          frame False {
            n271 = Enqueue Element(queue=w515, element=cluster{"命令":string, "data":variant} {"命令"="停用模块", "data"=variant} ("元素")) -> ()  [unwired: 2 in, 3 out]
          }
          frame True {
            n272 = Enqueue Element(queue=w517, element=cluster{"命令":string, "data":variant} {"命令"="启用模块", "data"=variant} ("元素")) -> ()  [unwired: 2 in, 3 out]
          }
        }
      }
      event "流程路径": Value Change {
        n273 = event-data() -> ()  [unwired: 1 in, 6 out]
        n274 = flat-sequence {
          frame #0 {
            n275 = local read "流程路径"() -> (w519:path)
            n276 = global write "氨氮断电保存全局变量.vi" "流程路径"(w519) -> ()
          }
          frame #1 {
            n277 = call <vilib>:"Application Directory.vi"() -> ("Application Directory"=w533:path)
            n278 = Build Path(base path=w533, name or relative path="data\\sys.ini" ("名称或相对路径")) -> (appended path=w531:path)
            n279 = call <vilib>:"Open Config Data.vi"("configuration file path"=w531) -> ("error out"=w527:errorcluster, "refnum"=w530:T13)  [unwired: 8 in, 1 out]
            n280 = vi-ref "氨氮断电保存全局变量.vi"() -> (w529:refnum<vi>)
            n281 = call <userlib>:"Write Panel to INI__ogtk.vi"("error in (no error)"=w527, "VI ref"=w529, "refnum"=w530) -> ("error out"=w526:errorcluster, "refnum out"=w528:T13)  [unwired: 7 in]
            n282 = call <vilib>:"Close Config Data.vi"("error in (no error)"=w526, "refnum"=w528) -> ("error out"=w521:errorcluster, "file path"=w520:path)  [unwired: 8 in]
            n283 = Open/Create/Replace File(file path (use dialog)=w520, error in=w521) -> (refnum out=w524:refnum<file>, error out=w525:errorcluster)  [unwired: 4 in, 1 out]
            n284 = Flush File(refnum=w524, error in=w525) -> (refnum out=w523:refnum<file>, error out=w522:errorcluster)
            n285 = Close File(refnum=w523, error in=w522) -> ()  [unwired: 2 out]
          }
        }
      }
      event "公式一键写入": Value Change {
        n286 = event-data() -> ()  [unwired: 1 in, 6 out]
        n287 = local read "公式"() -> (w534:cluster{"X^2":dbl, "X":dbl, "b":dbl})
        n288 = call "公式复合写入.vi"("公式"=w534) -> ()  [unwired: 11 in]
      }
      event "备用系数一键写入": Value Change {
        n289 = event-data() -> ()  [unwired: 1 in, 6 out]
        n290 = local read "备用系数"() -> (w535:T2)
        n291 = call "量程参数复合参数写入.vi"("备用系数"=w535) -> ()  [unwired: 11 in]
      }
      event "曲线模型": Value Change {
        n292 = event-data() -> ()  [unwired: 1 in, 6 out]
        n293 = local write "公式"("曲线模型") -> ()
      }
      event "质控参数设置": Value Change {
        n294 = event-data() -> ()  [unwired: 1 in, 6 out]
        n295 = global read "氨氮断电保存全局变量.vi" "质控参数设置"() -> (w537:T20)
        n296 = call "氨氮质控参数设置.vi"("质控参数设置"=w537) -> ("输出簇"=w538:T21)  [unwired: 10 in]
        n297 = Unbundle By Name(w538) -> ("确定"=w539:bool)
        n298 = case shown="真" w539 {
          tunnel: w538 -> [_ w541]
          tunnel: w537 -> [_ w540]
          frame False {
          }
          frame True {
            n299 = flat-sequence {
              tunnel: w541 -> [w548]
              tunnel: w540 -> [w547]
              frame #0 {
                n300 = Unbundle By Name(w548) -> ("跨度值"=w546:dbl, "零点标准液浓度"=w545:dbl, "跨度标准液浓度"=w544:dbl, "标准液标准浓度"=w543:dbl)
                n301 = Bundle By Name(cluster=w547, "氨氮跨度值"=w546, "氨氮零点标准液浓度"=w545, "氨氮跨度标准液浓度"=w544, "氨氮标准液标准浓度"=w543) -> (w542:T20)
                n302 = global write "氨氮断电保存全局变量.vi" "质控参数设置"(w542) -> ()
              }
              frame #1 {
                n303 = call <vilib>:"Application Directory.vi"() -> ("Application Directory"=w562:path)
                n304 = Build Path(base path=w562, name or relative path="data\\sys.ini" ("名称或相对路径")) -> (appended path=w560:path)
                n305 = call <vilib>:"Open Config Data.vi"("configuration file path"=w560) -> ("error out"=w556:errorcluster, "refnum"=w559:T13)  [unwired: 8 in, 1 out]
                n306 = vi-ref "氨氮断电保存全局变量.vi"() -> (w558:refnum<vi>)
                n307 = call <userlib>:"Write Panel to INI__ogtk.vi"("error in (no error)"=w556, "VI ref"=w558, "refnum"=w559) -> ("error out"=w555:errorcluster, "refnum out"=w557:T13)  [unwired: 7 in]
                n308 = call <vilib>:"Close Config Data.vi"("error in (no error)"=w555, "refnum"=w557) -> ("error out"=w550:errorcluster, "file path"=w549:path)  [unwired: 8 in]
                n309 = Open/Create/Replace File(file path (use dialog)=w549, error in=w550) -> (refnum out=w553:refnum<file>, error out=w554:errorcluster)  [unwired: 4 in, 1 out]
                n310 = Flush File(refnum=w553, error in=w554) -> (refnum out=w552:refnum<file>, error out=w551:errorcluster)
                n311 = Close File(refnum=w552, error in=w551) -> ()  [unwired: 2 out]
              }
            }
          }
        }
      }
      event "自动测试量程配置": Value Change {
        n312 = event-data() -> ()  [unwired: 1 in, 6 out]
        n313 = flat-sequence {
          frame #0 {
            n314 = global write "氨氮断电保存全局变量.vi" "氨氮自动测试量程配置"("自动测试量程配置") -> ()
          }
          frame #1 {
            n315 = call <vilib>:"Application Directory.vi"() -> ("Application Directory"=w577:path)
            n316 = Build Path(base path=w577, name or relative path="data\\sys.ini" ("名称或相对路径")) -> (appended path=w575:path)
            n317 = call <vilib>:"Open Config Data.vi"("configuration file path"=w575) -> ("error out"=w571:errorcluster, "refnum"=w574:T13)  [unwired: 8 in, 1 out]
            n318 = vi-ref "氨氮断电保存全局变量.vi"() -> (w573:refnum<vi>)
            n319 = call <userlib>:"Write Panel to INI__ogtk.vi"("error in (no error)"=w571, "VI ref"=w573, "refnum"=w574) -> ("error out"=w570:errorcluster, "refnum out"=w572:T13)  [unwired: 7 in]
            n320 = call <vilib>:"Close Config Data.vi"("error in (no error)"=w570, "refnum"=w572) -> ("error out"=w565:errorcluster, "file path"=w564:path)  [unwired: 8 in]
            n321 = Open/Create/Replace File(file path (use dialog)=w564, error in=w565) -> (refnum out=w568:refnum<file>, error out=w569:errorcluster)  [unwired: 4 in, 1 out]
            n322 = Flush File(refnum=w568, error in=w569) -> (refnum out=w567:refnum<file>, error out=w566:errorcluster)
            n323 = Close File(refnum=w567, error in=w566) -> ()  [unwired: 2 out]
          }
        }
      }
      event "手动启动": Value Change {
        n324 = event-data() -> ()  [unwired: 1 in, 6 out]
        n325 = call "氨氮启动参数对话框.vi"() -> ("确认"=w578:bool, "元素"=w579:cluster{"命令":string, "data":variant})  [unwired: 10 in]
        n326 = case shown="真" w578 {
          tunnel: w580 -> [_ w582]
          tunnel: w579 -> [_ w581]
          frame False {
          }
          frame True {
            n327 = Enqueue Element(queue=w582, element=w581) -> ()  [unwired: 2 in, 3 out]
          }
        }
      }
      event "定时启动": Mouse Down {
        n328 = event-data() -> ()  [unwired: 1 in, 6 out]
        n329 = flat-sequence {
          frame #0 {
            n330 = global read "氨氮断电保存全局变量.vi" "定时控制"() -> (w584:T6)
            n331 = call "周期设置.vi"("定时控制输入"=w584) -> ("定时控制输出"=w583:T22)  [unwired: 10 in]
            n332 = global write "氨氮断电保存全局变量.vi" "定时控制"(w583) -> ()
          }
          frame #1 {
            n333 = call <vilib>:"Application Directory.vi"() -> ("Application Directory"=w598:path)
            n334 = Build Path(base path=w598, name or relative path="data\\sys.ini" ("名称或相对路径")) -> (appended path=w596:path)
            n335 = call <vilib>:"Open Config Data.vi"("configuration file path"=w596) -> ("error out"=w592:errorcluster, "refnum"=w595:T13)  [unwired: 8 in, 1 out]
            n336 = vi-ref "氨氮断电保存全局变量.vi"() -> (w594:refnum<vi>)
            n337 = call <userlib>:"Write Panel to INI__ogtk.vi"("error in (no error)"=w592, "VI ref"=w594, "refnum"=w595) -> ("error out"=w591:errorcluster, "refnum out"=w593:T13)  [unwired: 7 in]
            n338 = call <vilib>:"Close Config Data.vi"("error in (no error)"=w591, "refnum"=w593) -> ("error out"=w586:errorcluster, "file path"=w585:path)  [unwired: 8 in]
            n339 = Open/Create/Replace File(file path (use dialog)=w585, error in=w586) -> (refnum out=w589:refnum<file>, error out=w590:errorcluster)  [unwired: 4 in, 1 out]
            n340 = Flush File(refnum=w589, error in=w590) -> (refnum out=w588:refnum<file>, error out=w587:errorcluster)
            n341 = Close File(refnum=w588, error in=w587) -> ()  [unwired: 2 out]
          }
        }
      }
      event "单步测试": Value Change {
        w600 = u16 1 items=["总磷"=1, "氨氮"=3] ("站号")
        n342 = event-data() -> ()  [unwired: 1 in, 6 out]
        n343 = Bundle("站号"=w600, "总磷氨氮调试"="总磷氨氮调试") -> (w599:cluster{"站号":u16, "总磷氨氮调试":u16[]})  [unwired: 1 in]
        n344 = Bundle By Name(cluster=cluster{"命令":string, "data":variant} {"命令"="", "data"=variant} ("元素"), "命令"="debug", "data"=w599) -> (w602:cluster{"命令":string, "data":variant})
        n345 = Enqueue Element(queue=w605, element=w602) -> ()  [unwired: 2 in, 3 out]
      }
      event "停止": Value Change {
        n346 = event-data() -> ()  [unwired: 1 in, 6 out]
        n347 = Enqueue Element(queue=w612, element=cluster{"命令":string, "data":variant} {"命令"="启动", "data"=variant(cluster{"站号":u16, "控制命令输出":u16[]} {"站号"=1, "控制命令输出"=[2816]})} ("元素")) -> (queue out=w609:refnum<queue>)  [unwired: 2 in, 2 out]
        n348 = Cancel Notification(0:w607) -> (8:w608:refnum<notifier>)  [unwired: 1 in, 2 out]
        n349 = Send Notification(notification=TRUE ("通知"), notifier=w608) -> ()  [unwired: 1 in, 2 out]
        n350 = Enqueue Element(queue=w609, element=cluster{"命令":string, "data":variant} {"命令"="启动", "data"=variant(cluster{"站号":u16, "控制命令输出":u16[]} {"站号"=2, "控制命令输出"=[2816]})} ("元素")) -> ()  [unwired: 2 in, 3 out]
      }
      event "设置": Value Change {
        n351 = event-data() -> ()  [unwired: 1 in, 6 out]
        n352 = property on="窗格" class="Pane"("Origin"=T11 {"Horizontal"=0, "Vertical"=628} ("原点")) -> ()  [unwired: 2 in, 2 out]
      }
      event "返回": Value Change {
        n353 = event-data() -> ()  [unwired: 1 in, 6 out]
        n354 = property on="窗格" class="Pane"("Origin"=T11 {"Horizontal"=0, "Vertical"=0} ("原点")) -> ()  [unwired: 2 in, 2 out]
      }
      event "公式.X^2", "公式.X", "公式.b", "量程切换阈值.阈值", "量程切换阈值.标液浓度", "备用系数.量程上限", "备用系数.量程下限", "备用系数.检出限", "备用系数.精度": Mouse Down {
        n355 = event-data() -> ("CtlRef"=w618:refnum<vi>)  [unwired: 1 in, 5 out]
        n356 = property class="DigNum (严格)"(reference=w618) -> (reference out=w616:refnum<vi>, "Value"=w617:dbl)  [unwired: 1 in, 1 out]
        n357 = call "数字键盘.vi"("OldNumber"=w617) -> ("NewNumber"=w615:dbl)
        n358 = property class="DigNum (严格)"(reference=w616, "Val(Sgnl)"=w615) -> ()  [unwired: 1 in, 2 out]
      }
      event "读公式": Value Change {
        n359 = event-data() -> ()  [unwired: 1 in, 6 out]
        n360 = property class="Enum (严格)"(reference=w626) -> ("Value"=w625:enum16{"总磷", "总氮", "氨氮"})  [unwired: 1 in, 2 out]
        n361 = property class="Enum (严格)"(reference=w627) -> ("Value"=w624:enum16{"水样测量", "零点核查", "跨度核查", "标样核查", "加标回收"})  [unwired: 1 in, 2 out]
        n362 = property class="Enum (严格)"(reference=w628) -> ("Value"=w623:enum16{"低量程", "高量程"})  [unwired: 1 in, 2 out]
        n363 = call "公式读取.vi"("量程"=w623, "测量模式"=w624, "测量参数"=w625) -> ("error out"=w620:errorcluster, "公式"=w621:cluster{"X^2":dbl, "X":dbl, "b":dbl})  [unwired: 7 in]
        n364 = property class="Clust (严格)"(reference=w622, "Value"=w621) -> ()  [unwired: 1 in, 2 out]
        n365 = case shown="错误" w620 {
          tunnel: ["读取成功" ("消息") "读取失败" ("消息")] -> w619
          frame No Error {
          }
          frame Error {
          }
        }
        n366 = One Button Dialog(message=w619) -> ()  [unwired: 1 in, 1 out]
      }
      event "写公式": Value Change {
        n367 = event-data() -> ()  [unwired: 1 in, 6 out]
        n368 = call "公式写入.vi"("公式"="公式", "量程"="量程下拉列表", "测量模式"="测量模式下拉列表", "测量参数"="参数下拉列表") -> ("error out"=w633:errorcluster)  [unwired: 7 in]
        n369 = case shown="无错误" w633 {
          tunnel: ["写入成功" ("消息") "写入失败" ("消息")] -> w634
          frame No Error {
          }
          frame Error {
          }
        }
        n370 = One Button Dialog(message=w634) -> ()  [unwired: 1 in, 1 out]
      }
      event "量程切换阈值读取": Value Change {
        n371 = event-data() -> ()  [unwired: 1 in, 6 out]
        n372 = property class="Enum (严格)"(reference=w646) -> ("Value"=w645:enum16{"总磷", "总氮", "氨氮"})  [unwired: 1 in, 2 out]
        n373 = property class="Enum (严格)"(reference=w647) -> ("Value"=w644:enum16{"水样测量", "零点核查", "跨度核查", "标样核查", "加标回收"})  [unwired: 1 in, 2 out]
        n374 = property class="Enum (严格)"(reference=w648) -> ("Value"=w643:enum16{"低量程", "高量程"})  [unwired: 1 in, 2 out]
        n375 = call "量程读取.vi"("量程"=w643, "测量模式"=w644, "测量参数"=w645) -> ("error out"=w639:errorcluster, "量程切换阈值"=w641:cluster{"阈值":dbl, "标液浓度":dbl})  [unwired: 7 in]
        n376 = property class="Clust (严格)"(reference=w642, "Value"=w641) -> ()  [unwired: 1 in, 2 out]
        n377 = case shown="错误" w639 {
          tunnel: ["读取成功" ("消息") "读取失败" ("消息")] -> w640
          frame No Error {
          }
          frame Error {
          }
        }
        n378 = One Button Dialog(message=w640) -> ()  [unwired: 1 in, 1 out]
      }
      event "量程切换阈值写入": Value Change {
        n379 = event-data() -> ()  [unwired: 1 in, 6 out]
        n380 = property class="Enum (严格)"(reference=w659) -> ("Value"=w656:enum16{"总磷", "总氮", "氨氮"})  [unwired: 1 in, 2 out]
        n381 = property class="Enum (严格)"(reference=w658) -> ("Value"=w655:enum16{"水样测量", "零点核查", "跨度核查", "标样核查", "加标回收"})  [unwired: 1 in, 2 out]
        n382 = property class="Enum (严格)"(reference=w657) -> ("Value"=w654:enum16{"低量程", "高量程"})  [unwired: 1 in, 2 out]
        n383 = call "量程写入.vi"("量程切换阈值"="量程切换阈值", "量程"=w654, "测量模式"=w655, "测量参数"=w656) -> ("error out"=w651:errorcluster)  [unwired: 7 in]
        n384 = case shown="无错误" w651 {
          tunnel: ["写入成功" ("消息") "写入失败" ("消息")] -> w652
          frame No Error {
          }
          frame Error {
          }
        }
        n385 = One Button Dialog(message=w652) -> ()  [unwired: 1 in, 1 out]
      }
      event "备用系数读取": Value Change {
        n386 = event-data() -> ()  [unwired: 1 in, 6 out]
        n387 = property class="Enum (严格)"(reference=w671) -> ("Value"=w670:enum16{"总磷", "总氮", "氨氮"})  [unwired: 1 in, 2 out]
        n388 = property class="Enum (严格)"(reference=w665) -> ("Value"=w664:enum16{"水样测量", "零点核查", "跨度核查", "标样核查", "加标回收"})  [unwired: 1 in, 2 out]
        n389 = property class="Enum (严格)"(reference=w663) -> ("Value"=w662:enum16{"低量程", "高量程"})  [unwired: 1 in, 2 out]
        n390 = call "备用系数读取.vi"("量程"=w662, "测量模式"=w664, "测量参数"=w670) -> ("error out"=w666:errorcluster, "备用系数"=w668:T2)  [unwired: 7 in]
        n391 = property class="Clust (严格)"(reference=w669, "Value"=w668) -> ()  [unwired: 1 in, 2 out]
        n392 = case shown="错误" w666 {
          tunnel: ["读取成功" ("消息") "读取失败" ("消息")] -> w667
          frame No Error {
          }
          frame Error {
          }
        }
        n393 = One Button Dialog(message=w667) -> ()  [unwired: 1 in, 1 out]
      }
      event "备用系数写入": Value Change {
        n394 = event-data() -> ()  [unwired: 1 in, 6 out]
        n395 = property class="Enum (严格)"(reference=w682) -> ("Value"=w681:enum16{"总磷", "总氮", "氨氮"})  [unwired: 1 in, 2 out]
        n396 = property class="Enum (严格)"(reference=w677) -> ("Value"=w676:enum16{"水样测量", "零点核查", "跨度核查", "标样核查", "加标回收"})  [unwired: 1 in, 2 out]
        n397 = property class="Enum (严格)"(reference=w675) -> ("Value"=w674:enum16{"低量程", "高量程"})  [unwired: 1 in, 2 out]
        n398 = call "备用系数写入.vi"("备用系数"="备用系数", "量程"=w674, "测量模式"=w676, "测量参数"=w681) -> ("error out"=w678:errorcluster)  [unwired: 7 in]
        n399 = case shown="无错误" w678 {
          tunnel: ["写入成功" ("消息") "写入失败" ("消息")] -> w679
          frame No Error {
          }
          frame Error {
          }
        }
        n400 = One Button Dialog(message=w679) -> ()  [unwired: 1 in, 1 out]
      }
    }
  }
